vi "Diff Parameter.vi"(5 "parameter old":T3, 7 "parameter new":T3, 10 "change type":T1, 11 "refresh items in":T4[](array[typedef])) -> (3 "refresh items out":T4[](array[typedef]))   [LabVIEW 2020, in "AIM MIL-STD-1553 System Explorer.lvlib" / "Implementation.lvlib" / "Refresh.lvlib"]
uses:
  Refresh.lvlib
  MCL Row.ctl
  Change Type.ctl
  Symbols.ctl
  Shared/Parameter Definition.ctl
  Name to Symbol.vi
  Scripting/Constants.vi
  Scripting/AIM MIL-STD-1553 Scripting.lvlib
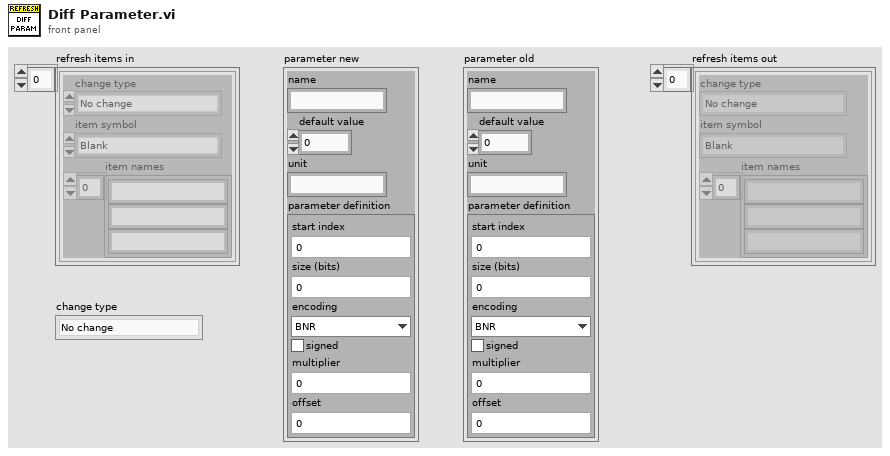
[diagram p1: front panel]
types:
  T1 = typedef "AIM MIL-STD-1553 System Explorer.lvlib/Implementation.lvlib/Refresh.lvlib/Change Type.ctl" = enum16{"No change", "Modify", "Add", "Remove"}
  T2 = typedef "Parameter Definition.ctl" = cluster{"start index":i32, "size (bits)":i32, "encoding":enum16{"BNR", "BCD", "Discrete"}, "signed":bool, "multiplier":dbl, "offset":dbl}
  T3 = cluster{"name":string, "default value":dbl, "unit":string, "parameter definition":T2}
  T4 = typedef "AIM MIL-STD-1553 System Explorer.lvlib/Implementation.lvlib/Refresh.lvlib/MCL Row.ctl" = cluster{"change type":T1, "item symbol":T5, "item names":string[]}
  T5 = typedef "AIM MIL-STD-1553 System Explorer.lvlib/Implementation.lvlib/Refresh.lvlib/Symbols.ctl" = enum16{"Blank", "MIL-STD-1553", "Port", "Remote Terminal", "Subaddress", "Bus Controller", "Frame", "Mode Code", "Message", "Parameter", "Item"}
  T6 = cluster{"name":string, "default value":string, "unit":string, "start index":string, "size":string, "encoding":string, "signed":string, "scale multiplier":string, "scale offset":string}
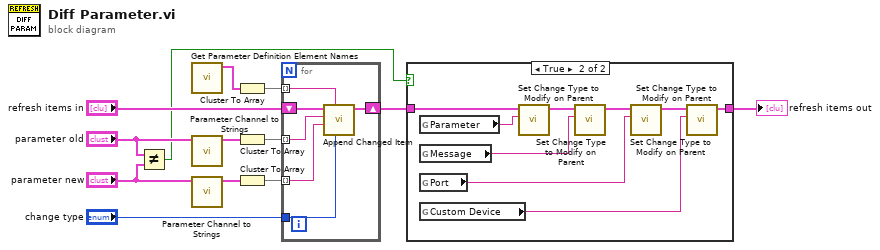
[diagram p0: block diagram]
diagram:
  n1 = Not Equal?(x="parameter old", y="parameter new") -> (x != y?=w8:bool)
  n2 = call "Get Parameter Definition Element Names.vi"() -> ("names"=w1:T6)  [unwired: 11 in]
  n3 = call "Parameter Channel to Strings.vi"("parameter channel definition"="parameter old") -> ("parameter channel strings"=w7:T6)  [unwired: 10 in]
  n4 = call "Parameter Channel to Strings.vi"("parameter channel definition"="parameter new") -> ("parameter channel strings"=w6:T6)  [unwired: 10 in]
  n5 = Cluster To Array(cluster=w1) -> (array=w2:string[])
  n6 = Cluster To Array(cluster=w7) -> (array=w4:string[])
  n7 = Cluster To Array(cluster=w6) -> (array=w3:string[])
  n8 = for {
    shift-right: [w18] -> w9
    shift-left: "refresh items in" -> [w19]
    tunnel: "change type" -> [w17]
    tunnel: w4 -> [w16] mode=indexing
    tunnel: w3 -> [w15] mode=indexing
    tunnel: w2 -> [w14] mode=indexing
    n9 = call "Append Changed Item.vi"("change type"=w17, "item name"=w14, "new value"=w15, "old value"=w16, "refresh items in"=w19) -> ("refresh items out"=w18:T4[])  [unwired: 5 in, 1 out]
  }
  n10 = case shown="True" w8 {
    tunnel: w9 -> [w20 w22]
    tunnel: [w20 w26] -> w13
    frame False {
    }
    frame True {
      n11 = global read "Constants.vi" "Parameter"() -> (w21:string)
      n12 = global read "Constants.vi" "Message"() -> (w28:string)
      n13 = global read "Constants.vi" "Port"() -> (w24:string)
      n14 = global read "Constants.vi" "Custom Device"() -> (w23:string)
      n15 = call "Set Change Type to Modify on Parent.vi"("parent name"=w21, "refresh items in"=w22) -> ()  [unwired: 9 in, 1 out]
      n16 = call "Set Change Type to Modify on Parent.vi"("parent name"=w28, "refresh items in"=w22) -> ("refresh items out"=w27:T4[])  [unwired: 9 in]
      n17 = call "Set Change Type to Modify on Parent.vi"("parent name"=w24, "refresh items in"=w27) -> ("refresh items out"=w25:T4[])  [unwired: 9 in]
      n18 = call "Set Change Type to Modify on Parent.vi"("parent name"=w23, "refresh items in"=w25) -> ("refresh items out"=w26:T4[])  [unwired: 9 in]
    }
  }
  "refresh items out" <- w13
